vi "flash_lamp (SubVI).vi"(9 "# Pulses in":i32) -> (3 "flash_out":dbl[](array[numeric]))   [LabVIEW 2014]
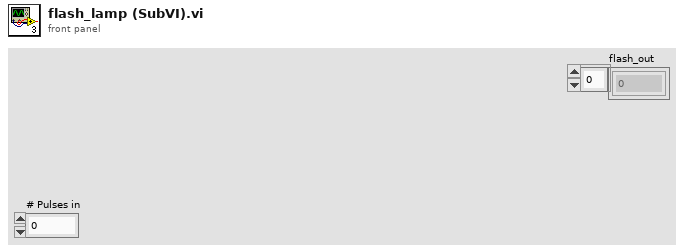
[diagram p1: front panel]
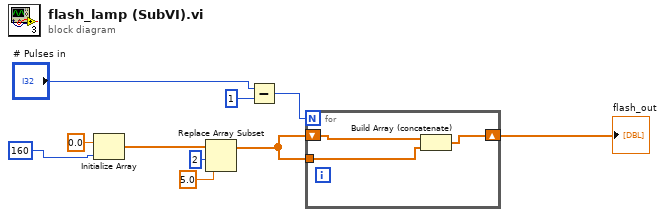
[diagram p0: block diagram]
diagram:
  n1 = Initialize Array(0.0 ("element"), 160 ("y")) -> (w2:dbl[])
  n2 = Replace Array Subset(array=w2, new element=5.0 ("new element/subarray"), index=2) -> (w7:dbl[])
  n3 = Subtract(x="# Pulses in", y=1) -> (x-y=w1:i32)
  n4 = for {
    N: w1 -> [_]
    shift-right: [w11] -> w3
    shift-left: w7 -> [w13]
    tunnel: w7 -> [w12]
    n5 = Build Array (concatenate)(w13, w12) -> (w11:dbl[])
  }
  "flash_out" <- w3
